vi "PH_VacuumControl.ProcCases.vi"(0 "i ref in":refnum<vi>, 1 "selector":string, 2 "Data":T1, 3 "call cluster":T2={"Object"="", "Selector"="", "CallType"=enum."synchronous", "Async Object"="", "Async Selector"="", "Data Descriptor"="", "Data"=[], "Error #"=0, "Expire"=0}, 5 "error in (no error)":errorcluster) -> (14 "i ref out":refnum<vi>, 17 "answer cluster":T2={"Object"="", "Selector"="", "CallType"=enum."synchronous", "Async Object"="", "Async Selector"="", "Data Descriptor"="", "Data"=[], "Error #"=0, "Expire"=0}, 19 "error out":errorcluster)   [LabVIEW 2014, in "PH_VacuumControl.lvlib"]
doc: "This method is called by a process from within the default case in the event loop. The methods of a class that are linked to events will be called from THIS method. Add your code here."
uses:
  PH_VacuumControl.lvlib
  CSCore/CSSystem/CoreDefs/CoreDefs.call_type.ctl
  CSCore/BaseProcess/BaseProcess.descriptor string definition.ctl
  CSCore/CSSystem/CoreDefs/CoreDefs.rawDataType.ctl
  CSCore/CSSystem/CoreLib/CoreLib.string 2 byte array.vi
  CSCore/CSSystem/CoreLib/CoreLib.byte array 2 double.vi
  CSCore/CSSystem/CoreLib/CoreLib.byte array 2 short.vi
  CSCore/CSSystem/CoreLib/CoreLib.byte array 2 int.vi
  CSCore/CSSystem/CoreLib/CoreLib.lvlib
  CSCore/BaseProcess/BaseProcess.lvlib
  instr.lib/AGCxxx/AGCxxx - Driver.lvlib
  CSCore/CAEObj/CAEObj.lvlib
  PH_PSDBWriter/PH_PSDBWriter.lvlib
  PH_Common/PH_Common.lvlib
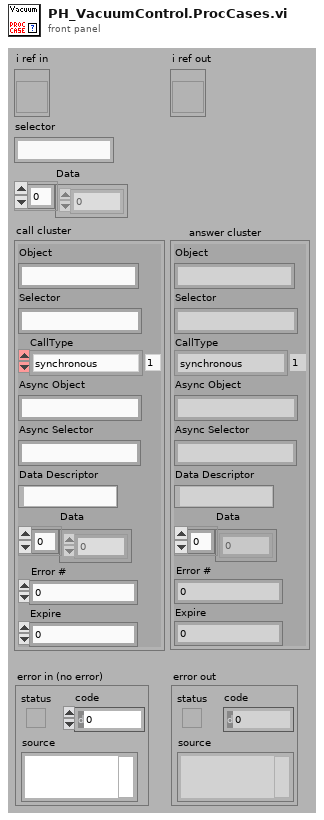
[diagram p1: front panel]
types:
  T1 = typedef "CoreDefs.rawDataType.ctl" = i8[]
  T2 = typedef "CoreDefs.call_type.ctl" = cluster{"Object":string, "Selector":string, "CallType":enum16{"simple", "synchronous", "asynchronous"}, "Async Object":string, "Async Selector":string, "Data Descriptor":T3, "Data":T1, "Error #":i32, "Expire":u32}
  T3 = typedef "BaseProcess.lvlib/BaseProcess.descriptor string definition.ctl" = string
  T4 = typedef "PH_VacuumControl.lvlib/PH_VacuumControl.i attribute.ctl" = cluster{"GUI Refs":cluster{"Exit":refnum<vi>, "Set Unit":refnum<vi>, "Device found":refnum<vi>, "Busy":refnum<vi>, "State":refnum<vi>, "Delete":refnum<vi>, "Channels":refnum<vi>, "Channel Name":refnum<vi>, "Trend":refnum<vi>, "Logarithmic":refnum<vi>, "Limit reached":refnum<vi>, "Channel Name 1 MT":refnum<vi>, "Channel Name 2 MT":refnum<vi>, "Trend MT":refnum<vi>, "Logarithmic MT":refnum<vi>, "Limit reached MT":refnum<vi>}, "Device found":bool, "Busy":bool, "Selected Unit":i32, "Channels [mbar]":T5, "Channel Names":cluster{"Channel 1":string, "Channel 2":string, "Channel 3":string, "Channel 4":string, "Channel 5":string, "Channel 6":string}, "Status":T6, "AGCxxx VISA Cluster":T7, "Instr Firmware Revision":string, "Service IDs Pressure":cluster{"Channel 1":i32, "Channel 2":i32, "Channel 3":i32, "Channel 4":i32, "Channel 5":i32, "Channel 6":i32}, "Service IDs Limits":cluster{"Channel 1":i32, "Channel 2":i32, "Channel 3":i32, "Channel 4":i32, "Channel 5":i32, "Channel 6":i32}, "Trend":cluster{"Start Point":timestamp, "Pressures [mbar] Channel 1":dbl[], "Pressures [mbar] Channel 2":dbl[], "Pressures [mbar] Channel 3":dbl[], "Pressures [mbar] Channel 4":dbl[], "Pressures [mbar] Channel 5":dbl[], "Pressures [mbar] Channel 6":dbl[], "Timebase [s]":i32[], "Trend Channel":u16, "Start Fit":dbl, "Trend Channel 1 MT":u16, "Trend Channel 2 MT":u16, "Start or continue Fit MT":dbl, "Continue or start Fit MT":dbl, "Datasets strored":i32, "Dataarray Size":i32}, "Running":bool}
  T5 = typedef "PH_VacuumControl.lvlib/PH_VacuumControl.Channels.ctl" = cluster{"Channel 1":dbl, "Channel 2":dbl, "Channel 3":dbl, "Channel 4":dbl, "Channel 5":dbl, "Channel 6":dbl, "Name Channel 1":string, "Name Channel 2":string, "Name Channel 3":string, "Name Channel 4":string, "Name Channel 5":string, "Name Channel 6":string, "Upper Limit":dbl, "Upper Limit 2":dbl, "Upper Limit 3":dbl, "Upper Limit 4":dbl, "Upper Limit 5":dbl, "Upper Limit 6":dbl}
  T6 = typedef "PH_StatusHandler.lvlib/PH_StatusHandler.Status.ctl" = i16
  T7 = typedef "AGCxxx - Driver.lvlib/AGCxxx VISA Control.ctl" = cluster{"VISA resource name":refnum<visa-resource-name>, "VISA Timeout Value (1000 ms)":u32, "Lock Timeout (1000 ms)":u32, "MAX Channel (6)":i32}
  T8 = typedef "PH_PSDBWriter.lvlib/PH_PSDBWriter.PHELIX-Subsystems.ctl" = i32
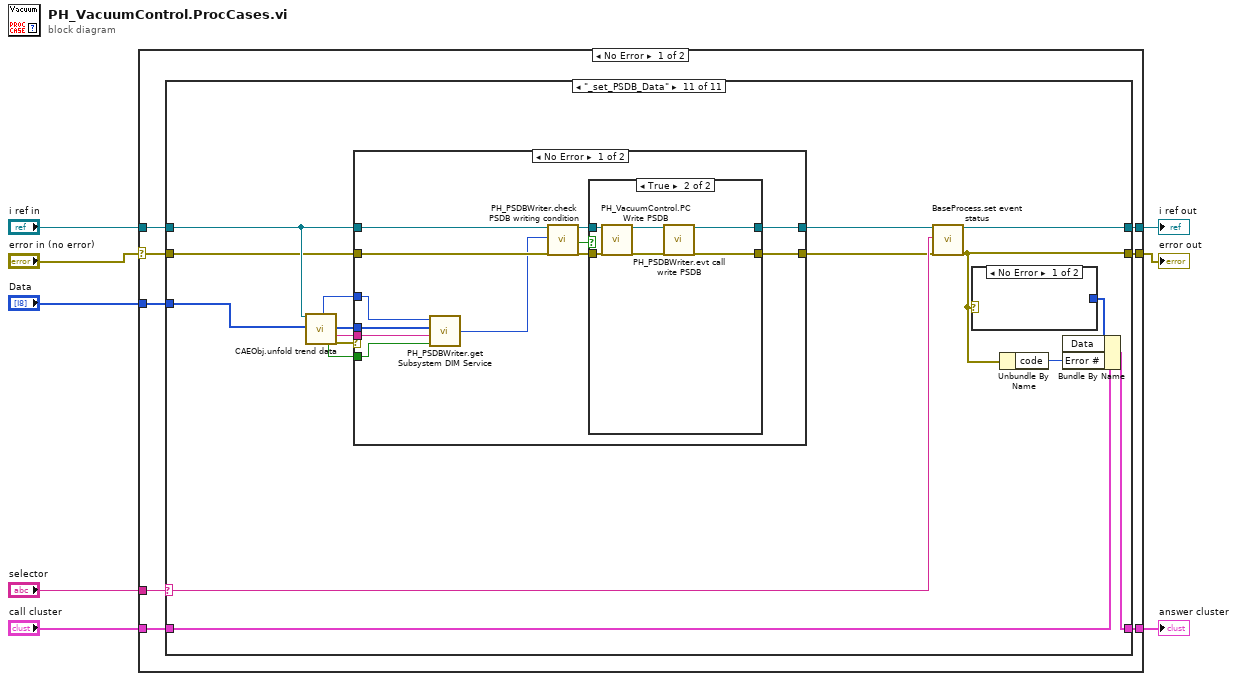
[diagram p0: block diagram]
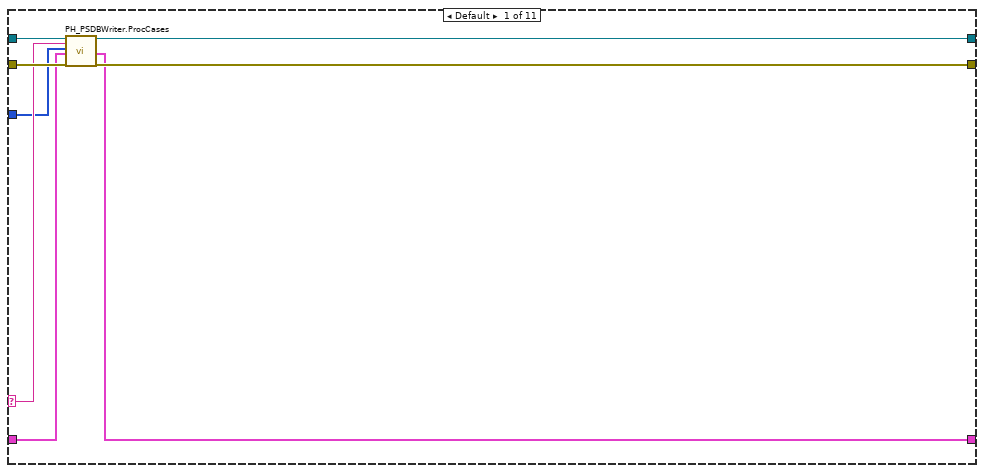
[diagram p2: hidden frame]
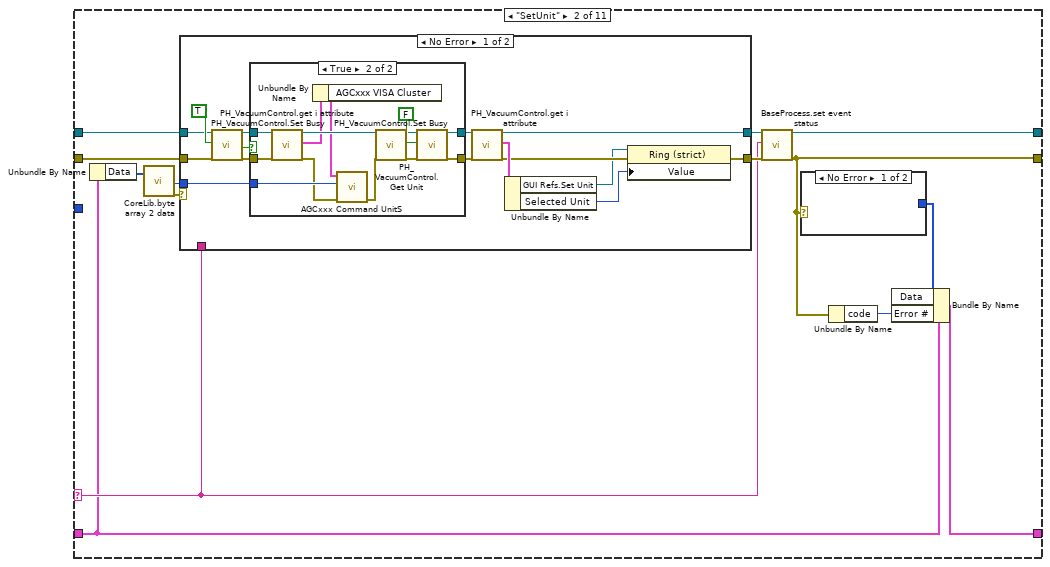
[diagram p3: hidden frame]
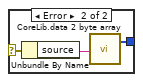
[diagram p4: hidden frame]
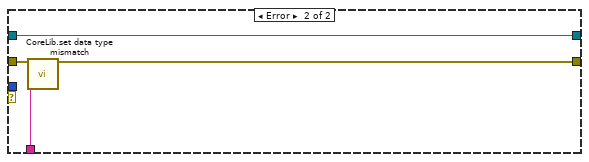
[diagram p6: hidden frame]
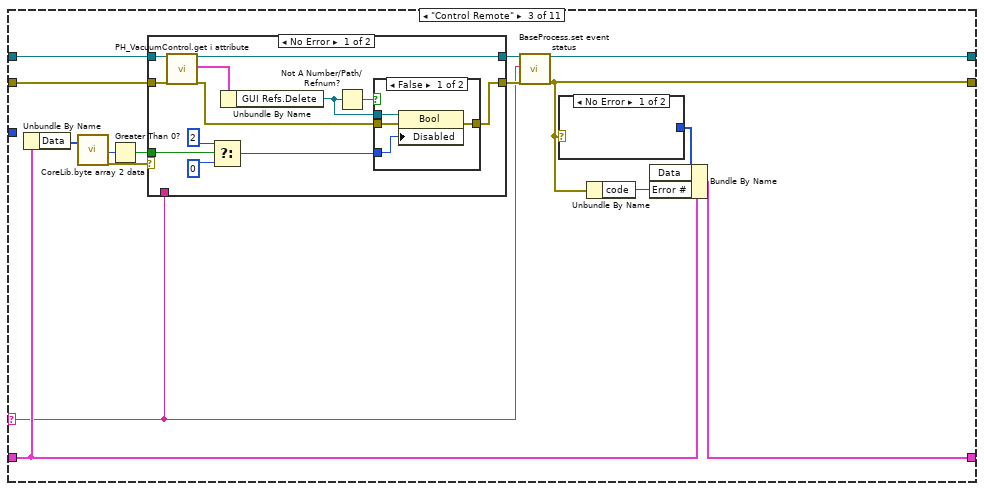
[diagram p7: hidden frame]
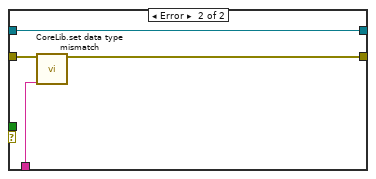
[diagram p9: hidden frame]
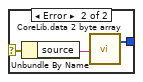
[diagram p10: hidden frame]
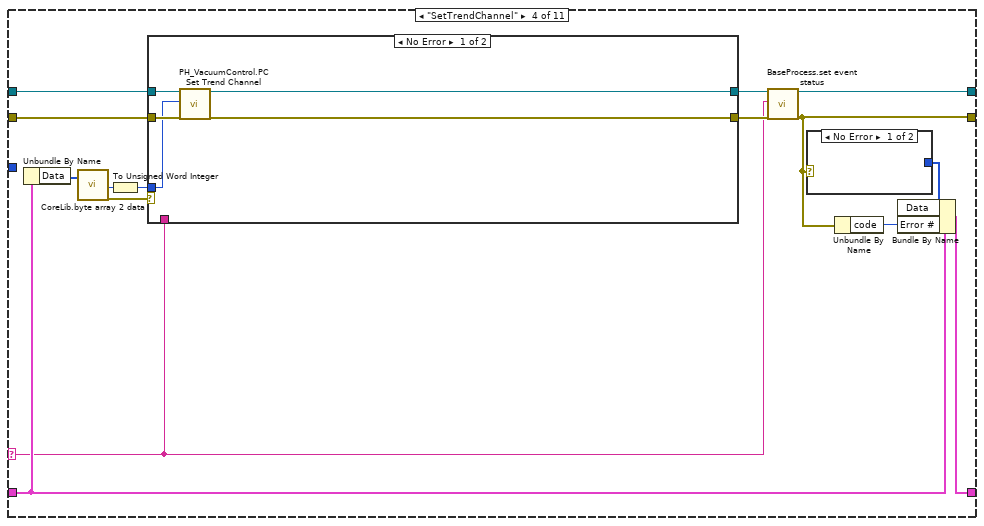
[diagram p11: hidden frame]
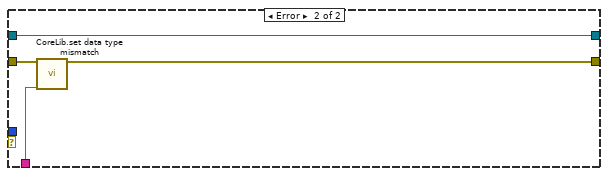
[diagram p12: hidden frame]
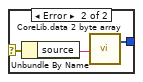
[diagram p13: hidden frame]
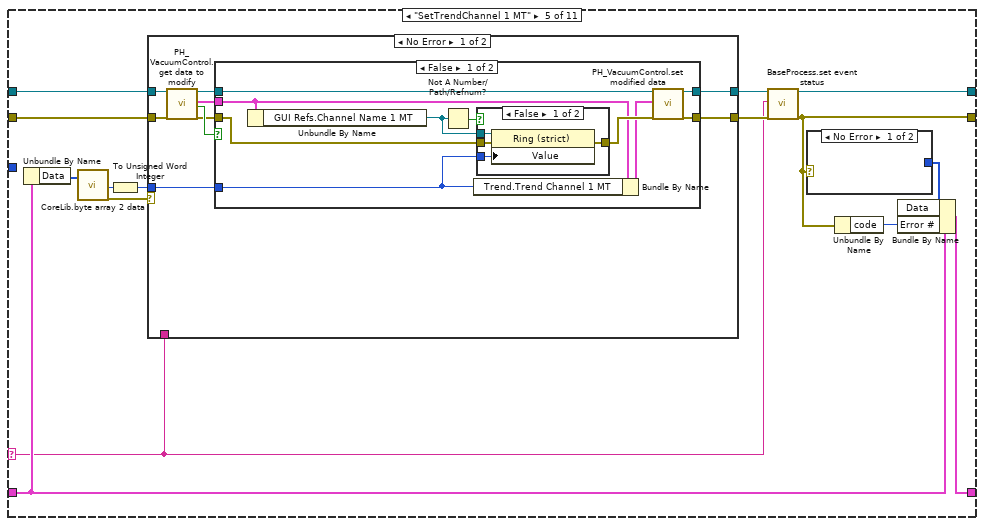
[diagram p14: hidden frame]
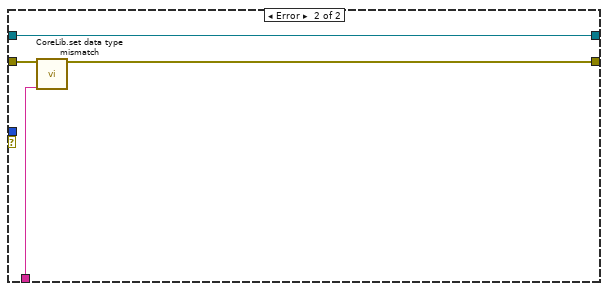
[diagram p17: hidden frame]
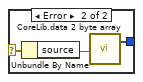
[diagram p18: hidden frame]
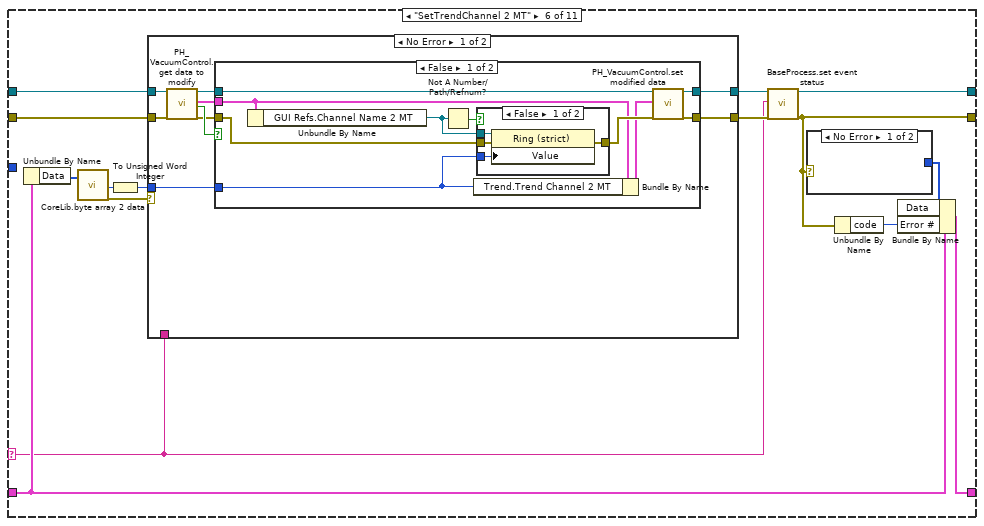
[diagram p19: hidden frame]
diagram:
  n1 = case shown="No Error" "error in (no error)" {
    selector: "error in (no error)" -> [w9 w431]
    tunnel: "selector" -> [w16 _]
    tunnel: [w15 w430] -> w7
    tunnel: "call cluster" -> [w14 w430]
    tunnel: "i ref in" -> [w13 w432]
    tunnel: [w12 w432] -> w4
    tunnel: [w11 w431] -> w3
    tunnel: "Data" -> [w10 _]
    frame No Error {
      n2 = case shown="\"_set_PSDB_Data\"" w16 {
        selector: w16 -> [w19 w27 w77 w116 w143 w191 w240 w267 w306 w349 w398]
        tunnel: w13 -> [w18 w38 w79 w118 w145 w193 w242 w269 w308 w351 w392]
        tunnel: [w24 w29 w88 w127 w154 w202 w250 w277 w316 w358 w402] -> w12
        tunnel: w14 -> [w20 w26 w83 w122 w149 w197 w246 w273 w312 w354 w399]
        tunnel: [w21 w25 w86 w125 w152 w200 w248 w275 w314 w356 w400] -> w15
        tunnel: w9 -> [w23 w37 w81 w120 w147 w195 w244 w271 w310 w353 w391]
        tunnel: [w22 w28 w87 w126 w153 w201 w249 w276 w315 w357 w401] -> w11
        tunnel: w10 -> [w17 _ _ _ _ _ _ _ _ _ w388]
        frame Default {
          n3 = call "PH_PSDBWriter.ProcCases.vi"("i ref in"=w18, "selector"=w19, "Data"=w17, "call cluster"=w20, "error in"=w23) -> ("i ref out"=w24:refnum<vi>, "answer cluster"=w21:T2, "error out"=w22:errorcluster)  [unwired: 12 in]
        }
        frame "SetUnit" {
          n4 = Unbundle By Name(w26) -> ("Data"=w36:T1)
          n5 = call-poly "CoreLib.byte array 2 data.vi"("byteArray"=w36) -> ("i32"=w34:i32, "error out"=w35:errorcluster)  [unwired: 16 in, 1 out]
          n6 = case shown="No Error" w35 {
            tunnel: [w49 w75] -> w30
            tunnel: w38 -> [w51 w75]
            tunnel: w37 -> [w52 w74]
            tunnel: [w44 w73] -> w31
            tunnel: w27 -> [_ w72]
            tunnel: w34 -> [w50 _]
            frame No Error {
              n7 = call "PH_VacuumControl.Set Busy.vi"("i ref in"=w51, "Busy"=TRUE, "error in (no error)"=w52) -> ("i ref out"=w54:refnum<vi>, "changed"=w53:bool, "error out"=w55:errorcluster)  [unwired: 14 in]
              n8 = case shown="True" w53 {
                tunnel: [w57 w70] -> w47
                tunnel: [w58 w69] -> w48
                tunnel: w55 -> [w57 w64]
                tunnel: w54 -> [w58 w66]
                tunnel: w50 -> [_ w61]
                frame False {
                }
                frame True {
                  n9 = call "PH_VacuumControl.get i attribute.vi"("i ref in"=w66, "error in (no error)"=w64) -> ("i ref out"=w65:refnum<vi>, "i attribute"=w63:T4, "error out"=w60:errorcluster)  [unwired: 15 in]
                  n10 = Unbundle By Name(w63) -> ("AGCxxx VISA Cluster"=w62:T7)
                  n11 = call "AGCxxx Command UnitS.vi"("error in (no error)"=w60, "unit (mBar)"=w61, "AGCxxx VISA Cluster"=w62) -> ("error out"=w59:errorcluster)  [unwired: 5 in, 2 out]
                  n12 = call "PH_VacuumControl.Get Unit.vi"("i ref in"=w65, "error in (no error)"=w59) -> ("i ref out"=w68:refnum<vi>, "error out"=w67:errorcluster)  [unwired: 16 in]
                  n13 = call "PH_VacuumControl.Set Busy.vi"("i ref in"=w68, "Busy"=FALSE, "error in (no error)"=w67) -> ("i ref out"=w69:refnum<vi>, "error out"=w70:errorcluster)  [unwired: 14 in, 1 out]
                }
              }
              n14 = call "PH_VacuumControl.get i attribute.vi"("i ref in"=w48, "error in (no error)"=w47) -> ("i ref out"=w49:refnum<vi>, "i attribute"=w46:T4, "error out"=w45:errorcluster)  [unwired: 15 in]
              n15 = Unbundle By Name(w46) -> ("GUI Refs.Set Unit"=w43:refnum<vi>, "Selected Unit"=w42:i32)
              n16 = property class="Ring (strict)"(reference=w43, error in=w45, "Value"=w42) -> (error out=w44:errorcluster)  [unwired: 1 out]
            }
            frame Error {
              n17 = call "CoreLib.set data type mismatch.vi"("error in (no error)"=w74, "error source"=w72) -> ("error out"=w73:errorcluster)  [unwired: 17 in]
            }
          }
          n18 = call "BaseProcess.set event status.vi"("i ref in"=w30, "EventStatus"=w27, "error in (no error)"=w31) -> ("i ref out"=w29:refnum<vi>, "error out"=w28:errorcluster)  [unwired: 14 in, 1 out]
          n19 = case shown="No Error" w28 {
            selector: w28 -> [_ w41]
            tunnel: [_ w39] -> w32
            frame No Error {
            }
            frame Error {
              n20 = Unbundle By Name(w41) -> ("source"=w40:string)
              n21 = call-poly "CoreLib.data 2 byte array.vi"("string"=w40) -> ("byteArray out"=w39:T1)  [unwired: 18 in]
            }
          }
          n22 = Unbundle By Name(w28) -> ("code"=w33:i32)
          n23 = Bundle By Name(cluster=w26, "Data"=w32, "Error #"=w33) -> (w25:T2)
        }
        frame "Control Remote" {
          n24 = Unbundle By Name(w83) -> ("Data"=w85:T1)
          n25 = call-poly "CoreLib.byte array 2 data.vi"("byteArray"=w85) -> ("i16"=w84:i16, "error out"=w82:errorcluster)  [unwired: 16 in, 1 out]
          n26 = Greater Than 0?(x=w84) -> (x > 0?=w76:bool)
          n27 = case shown="No Error" w82 {
            tunnel: w81 -> [w101 w111]
            tunnel: [w98 w110] -> w80
            tunnel: w79 -> [w102 w109]
            tunnel: [w100 w109] -> w78
            tunnel: w77 -> [_ w108]
            tunnel: w76 -> [w94 _]
            frame No Error {
              n28 = call "PH_VacuumControl.get i attribute.vi"("i ref in"=w102, "error in (no error)"=w101) -> ("i ref out"=w100:refnum<vi>, "i attribute"=w99:T4, "error out"=w97:errorcluster)  [unwired: 15 in]
              n29 = Select(t=u8 2 ("Disabled"), s=w94, f=u8 0 ("Disabled")) -> (s? t:f=w93:u8)
              n30 = Unbundle By Name(w99) -> ("GUI Refs.Delete"=w96:refnum<vi>)
              n31 = Not A Number/Path/Refnum?(number/path/refnum=w96) -> (NaN/Path/Refnum?=w95:bool)
              n32 = case shown="False" w95 {
                tunnel: [w106 w107] -> w98
                tunnel: w97 -> [w105 w107]
                tunnel: w96 -> [w104 _]
                tunnel: w93 -> [w103 _]
                frame False {
                  n33 = property class="Bool"(reference=w104, error in=w105, "Disabled"=w103) -> (error out=w106:errorcluster)  [unwired: 1 out]
                }
                frame True {
                }
              }
            }
            frame Error {
              n34 = call "CoreLib.set data type mismatch.vi"("error in (no error)"=w111, "error source"=w108) -> ("error out"=w110:errorcluster)  [unwired: 17 in]
            }
          }
          n35 = call "BaseProcess.set event status.vi"("i ref in"=w78, "EventStatus"=w77, "error in (no error)"=w80) -> ("i ref out"=w88:refnum<vi>, "error out"=w87:errorcluster)  [unwired: 14 in, 1 out]
          n36 = case shown="No Error" w87 {
            selector: w87 -> [_ w114]
            tunnel: [_ w112] -> w89
            frame No Error {
            }
            frame Error {
              n37 = Unbundle By Name(w114) -> ("source"=w113:string)
              n38 = call-poly "CoreLib.data 2 byte array.vi"("string"=w113) -> ("byteArray out"=w112:T1)  [unwired: 18 in]
            }
          }
          n39 = Unbundle By Name(w87) -> ("code"=w90:i32)
          n40 = Bundle By Name(cluster=w83, "Data"=w89, "Error #"=w90) -> (w86:T2)
        }
        frame "SetTrendChannel" {
          n41 = Unbundle By Name(w122) -> ("Data"=w124:T1)
          n42 = call-poly "CoreLib.byte array 2 data.vi"("byteArray"=w124) -> ("i16"=w123:i16, "error out"=w121:errorcluster)  [unwired: 16 in, 1 out]
          n43 = To Unsigned Word Integer(number=w123) -> (unsigned 16bit integer=w115:u16)
          n44 = case shown="No Error" w121 {
            tunnel: w120 -> [w133 w138]
            tunnel: [w132 w137] -> w119
            tunnel: w118 -> [w134 w136]
            tunnel: [w131 w136] -> w117
            tunnel: w116 -> [_ w135]
            tunnel: w115 -> [w130 _]
            frame No Error {
              n45 = call "PH_VacuumControl.PC Set Trend Channel.vi"("i ref in"=w134, "Trend Channel"=w130, "error IO"=w133) -> ("i ref out"=w131:refnum<vi>, "error out"=w132:errorcluster)  [unwired: 15 in]
            }
            frame Error {
              n46 = call "CoreLib.set data type mismatch.vi"("error in (no error)"=w138, "error source"=w135) -> ("error out"=w137:errorcluster)  [unwired: 17 in]
            }
          }
          n47 = call "BaseProcess.set event status.vi"("i ref in"=w117, "EventStatus"=w116, "error in (no error)"=w119) -> ("i ref out"=w127:refnum<vi>, "error out"=w126:errorcluster)  [unwired: 14 in, 1 out]
          n48 = case shown="No Error" w126 {
            selector: w126 -> [_ w141]
            tunnel: [_ w139] -> w128
            frame No Error {
            }
            frame Error {
              n49 = Unbundle By Name(w141) -> ("source"=w140:string)
              n50 = call-poly "CoreLib.data 2 byte array.vi"("string"=w140) -> ("byteArray out"=w139:T1)  [unwired: 18 in]
            }
          }
          n51 = Unbundle By Name(w126) -> ("code"=w129:i32)
          n52 = Bundle By Name(cluster=w122, "Data"=w128, "Error #"=w129) -> (w125:T2)
        }
        frame "SetTrendChannel 1 MT" {
          n53 = Unbundle By Name(w149) -> ("Data"=w151:T1)
          n54 = call-poly "CoreLib.byte array 2 data.vi"("byteArray"=w151) -> ("i16"=w150:i16, "error out"=w148:errorcluster)  [unwired: 16 in, 1 out]
          n55 = To Unsigned Word Integer(number=w150) -> (unsigned 16bit integer=w142:u16)
          n56 = case shown="No Error" w148 {
            tunnel: w147 -> [w160 w186]
            tunnel: [w158 w185] -> w146
            tunnel: w145 -> [w161 w184]
            tunnel: [w159 w184] -> w144
            tunnel: w143 -> [_ w183]
            tunnel: w142 -> [w157 _]
            frame No Error {
              n57 = call "PH_VacuumControl.get data to modify.vi"("i ref in"=w161, "error in (no error)"=w160) -> ("i ref out"=w165:refnum<vi>, "i attribute"=w162:T4, "timed out"=w164:bool, "error out"=w163:errorcluster)  [unwired: 14 in]
              n58 = case shown="False" w164 {
                tunnel: w162 -> [w168 _]
                tunnel: w163 -> [w174 w181]
                tunnel: [w171 w181] -> w158
                tunnel: w165 -> [w170 w182]
                tunnel: [w169 w182] -> w159
                tunnel: w157 -> [w166 _]
                frame False {
                  n59 = Unbundle By Name(w168) -> ("GUI Refs.Channel Name 1 MT"=w173:refnum<vi>)
                  n60 = Not A Number/Path/Refnum?(number/path/refnum=w173) -> (NaN/Path/Refnum?=w172:bool)
                  n61 = Bundle By Name(cluster=w168, "Trend.Trend Channel 1 MT"=w166) -> (w167:T4)
                  n62 = case shown="False" w172 {
                    tunnel: [w179 w180] -> w175
                    tunnel: w174 -> [w178 w180]
                    tunnel: w173 -> [w177 _]
                    tunnel: w166 -> [w176 _]
                    frame False {
                      n63 = property class="Ring (strict)"(reference=w177, error in=w178, "Value"=w176) -> (error out=w179:errorcluster)  [unwired: 1 out]
                    }
                    frame True {
                    }
                  }
                  n64 = call "PH_VacuumControl.set modified data.vi"("i ref in"=w170, "i attribute"=w167, "error in (no error)"=w175) -> ("i ref out"=w169:refnum<vi>, "error out"=w171:errorcluster)  [unwired: 15 in]
                }
                frame True {
                }
              }
            }
            frame Error {
              n65 = call "CoreLib.set data type mismatch.vi"("error in (no error)"=w186, "error source"=w183) -> ("error out"=w185:errorcluster)  [unwired: 17 in]
            }
          }
          n66 = call "BaseProcess.set event status.vi"("i ref in"=w144, "EventStatus"=w143, "error in (no error)"=w146) -> ("i ref out"=w154:refnum<vi>, "error out"=w153:errorcluster)  [unwired: 14 in, 1 out]
          n67 = case shown="No Error" w153 {
            selector: w153 -> [_ w189]
            tunnel: [_ w187] -> w155
            frame No Error {
            }
            frame Error {
              n68 = Unbundle By Name(w189) -> ("source"=w188:string)
              n69 = call-poly "CoreLib.data 2 byte array.vi"("string"=w188) -> ("byteArray out"=w187:T1)  [unwired: 18 in]
            }
          }
          n70 = Unbundle By Name(w153) -> ("code"=w156:i32)
          n71 = Bundle By Name(cluster=w149, "Data"=w155, "Error #"=w156) -> (w152:T2)
        }
        frame "SetTrendChannel 2 MT" {
          n72 = Unbundle By Name(w197) -> ("Data"=w199:T1)
          n73 = call-poly "CoreLib.byte array 2 data.vi"("byteArray"=w199) -> ("i16"=w198:i16, "error out"=w196:errorcluster)  [unwired: 16 in, 1 out]
          n74 = To Unsigned Word Integer(number=w198) -> (unsigned 16bit integer=w190:u16)
          n75 = case shown="No Error" w196 {
            tunnel: w195 -> [w208 w234]
            tunnel: [w206 w233] -> w194
            tunnel: w193 -> [w209 w232]
            tunnel: [w207 w232] -> w192
            tunnel: w191 -> [_ w231]
            tunnel: w190 -> [w205 _]
            frame No Error {
              n76 = call "PH_VacuumControl.get data to modify.vi"("i ref in"=w209, "error in (no error)"=w208) -> ("i ref out"=w213:refnum<vi>, "i attribute"=w210:T4, "timed out"=w212:bool, "error out"=w211:errorcluster)  [unwired: 14 in]
              n77 = case shown="False" w212 {
                tunnel: w210 -> [w216 _]
                tunnel: w211 -> [w222 w229]
                tunnel: [w219 w229] -> w206
                tunnel: w213 -> [w218 w230]
                tunnel: [w217 w230] -> w207
                tunnel: w205 -> [w214 _]
                frame False {
                  n78 = Unbundle By Name(w216) -> ("GUI Refs.Channel Name 2 MT"=w221:refnum<vi>)
                  n79 = Not A Number/Path/Refnum?(number/path/refnum=w221) -> (NaN/Path/Refnum?=w220:bool)
                  n80 = Bundle By Name(cluster=w216, "Trend.Trend Channel 2 MT"=w214) -> (w215:T4)
                  n81 = case shown="False" w220 {
                    tunnel: [w227 w228] -> w223
                    tunnel: w222 -> [w226 w228]
                    tunnel: w221 -> [w225 _]
                    tunnel: w214 -> [w224 _]
                    frame False {
                      n82 = property class="Ring (strict)"(reference=w225, error in=w226, "Value"=w224) -> (error out=w227:errorcluster)  [unwired: 1 out]
                    }
                    frame True {
                    }
                  }
                  n83 = call "PH_VacuumControl.set modified data.vi"("i ref in"=w218, "i attribute"=w215, "error in (no error)"=w223) -> ("i ref out"=w217:refnum<vi>, "error out"=w219:errorcluster)  [unwired: 15 in]
                }
                frame True {
                }
              }
            }
            frame Error {
              n84 = call "CoreLib.set data type mismatch.vi"("error in (no error)"=w234, "error source"=w231) -> ("error out"=w233:errorcluster)  [unwired: 17 in]
            }
          }
          n85 = call "BaseProcess.set event status.vi"("i ref in"=w192, "EventStatus"=w191, "error in (no error)"=w194) -> ("i ref out"=w202:refnum<vi>, "error out"=w201:errorcluster)  [unwired: 14 in, 1 out]
          n86 = case shown="No Error" w201 {
            selector: w201 -> [_ w237]
            tunnel: [_ w235] -> w203
            frame No Error {
            }
            frame Error {
              n87 = Unbundle By Name(w237) -> ("source"=w236:string)
              n88 = call-poly "CoreLib.data 2 byte array.vi"("string"=w236) -> ("byteArray out"=w235:T1)  [unwired: 18 in]
            }
          }
          n89 = Unbundle By Name(w201) -> ("code"=w204:i32)
          n90 = Bundle By Name(cluster=w197, "Data"=w203, "Error #"=w204) -> (w200:T2)
        }
        frame "SetLogarithmic" {
          n91 = Unbundle By Name(w246) -> ("Data"=w247:T1)
          n92 = call-poly "CoreLib.byte array 2 data.vi"("byteArray"=w247) -> ("i16"=w239:i16, "error out"=w245:errorcluster)  [unwired: 16 in, 1 out]
          n93 = Greater Than 0?(x=w239) -> (x > 0?=w238:bool)
          n94 = case shown="No Error" w245 {
            tunnel: w244 -> [w256 w261]
            tunnel: [w254 w260] -> w243
            tunnel: w242 -> [w257 w259]
            tunnel: [w255 w259] -> w241
            tunnel: w240 -> [_ w258]
            tunnel: w238 -> [w253 _]
            frame No Error {
              n95 = call "PH_VacuumControl.PC Set Logarithmic.vi"("i ref in"=w257, "Logarithmic"=w253, "error IO"=w256) -> ("i ref out"=w255:refnum<vi>, "error out"=w254:errorcluster)  [unwired: 15 in]
            }
            frame Error {
              n96 = call "CoreLib.set data type mismatch.vi"("error in (no error)"=w261, "error source"=w258) -> ("error out"=w260:errorcluster)  [unwired: 17 in]
            }
          }
          n97 = call "BaseProcess.set event status.vi"("i ref in"=w241, "EventStatus"=w240, "error in (no error)"=w243) -> ("i ref out"=w250:refnum<vi>, "error out"=w249:errorcluster)  [unwired: 14 in, 1 out]
          n98 = case shown="No Error" w249 {
            selector: w249 -> [_ w264]
            tunnel: [_ w262] -> w251
            frame No Error {
            }
            frame Error {
              n99 = Unbundle By Name(w264) -> ("source"=w263:string)
              n100 = call-poly "CoreLib.data 2 byte array.vi"("string"=w263) -> ("byteArray out"=w262:T1)  [unwired: 18 in]
            }
          }
          n101 = Unbundle By Name(w249) -> ("code"=w252:i32)
          n102 = Bundle By Name(cluster=w246, "Data"=w251, "Error #"=w252) -> (w248:T2)
        }
        frame "SetMTLogarithmic" {
          n103 = Unbundle By Name(w273) -> ("Data"=w274:T1)
          n104 = call-poly "CoreLib.byte array 2 data.vi"("byteArray"=w274) -> ("i16"=w266:i16, "error out"=w272:errorcluster)  [unwired: 16 in, 1 out]
          n105 = Greater Than 0?(x=w266) -> (x > 0?=w265:bool)
          n106 = case shown="No Error" w272 {
            tunnel: w271 -> [w284 w301]
            tunnel: [w281 w300] -> w270
            tunnel: w269 -> [w283 w299]
            tunnel: [w282 w299] -> w268
            tunnel: w267 -> [_ w298]
            tunnel: w265 -> [w280 _]
            frame No Error {
              n107 = call "PH_VacuumControl.get i attribute.vi"("i ref in"=w283, "error in (no error)"=w284) -> ("i ref out"=w282:refnum<vi>, "i attribute"=w287:T4, "error out"=w288:errorcluster)  [unwired: 15 in]
              n108 = Unbundle By Name(w287) -> ("GUI Refs.Logarithmic MT"=w292:refnum<vi>, "GUI Refs.Trend MT"=w289:refnum<vi>)
              n109 = Boolean To (0,1)(Boolean=w280) -> (0, 1=w286:i16)
              n110 = To Unsigned Byte Integer(number=w286) -> (unsigned 8bit integer=w285:u8)
              n111 = Not A Number/Path/Refnum?(number/path/refnum=w289) -> (NaN/Path/Refnum?=w290:bool)
              n112 = case shown="False" w290 {
                tunnel: w285 -> [w296 _]
                tunnel: w289 -> [w295 _]
                tunnel: w288 -> [w294 w297]
                tunnel: [w293 w297] -> w291
                frame False {
                  n113 = property class="XYGraph (strict)"(reference=w295, error in=w294, "YScale.Mapping Mode"=w296) -> (error out=w293:errorcluster)  [unwired: 1 out]
                }
                frame True {
                }
              }
              n114 = call "PH_GUI.set boolean GUI object.vi"("Boolean Knob GUI Ref"=w292, "Value"=w280, "error in (no error)"=w291) -> ("error out"=w281:errorcluster)  [unwired: 16 in]
            }
            frame Error {
              n115 = call "CoreLib.set data type mismatch.vi"("error in (no error)"=w301, "error source"=w298) -> ("error out"=w300:errorcluster)  [unwired: 17 in]
            }
          }
          n116 = call "BaseProcess.set event status.vi"("i ref in"=w268, "EventStatus"=w267, "error in (no error)"=w270) -> ("i ref out"=w277:refnum<vi>, "error out"=w276:errorcluster)  [unwired: 14 in, 1 out]
          n117 = case shown="No Error" w276 {
            selector: w276 -> [_ w304]
            tunnel: [_ w302] -> w278
            frame No Error {
            }
            frame Error {
              n118 = Unbundle By Name(w304) -> ("source"=w303:string)
              n119 = call-poly "CoreLib.data 2 byte array.vi"("string"=w303) -> ("byteArray out"=w302:T1)  [unwired: 18 in]
            }
          }
          n120 = Unbundle By Name(w276) -> ("code"=w279:i32)
          n121 = Bundle By Name(cluster=w273, "Data"=w278, "Error #"=w279) -> (w275:T2)
        }
        frame "SetFitStart" {
          n122 = Unbundle By Name(w312) -> ("Data"=w313:T1)
          n123 = call-poly "CoreLib.byte array 2 data.vi"("byteArray"=w313) -> ("d64"=w305:dbl, "error out"=w311:errorcluster)  [unwired: 16 in, 1 out]
          n124 = case shown="No Error" w311 {
            tunnel: w310 -> [w326 w340]
            tunnel: [w322 w339] -> w309
            tunnel: w308 -> [w327 w338]
            tunnel: [w324 w338] -> w307
            tunnel: w306 -> [_ w337]
            tunnel: w305 -> [w319 _]
            frame No Error {
              n125 = call "PH_VacuumControl.get data to modify.vi"("i ref in"=w327, "error in (no error)"=w326) -> ("i ref out"=w325:refnum<vi>, "i attribute"=w320:T4, "timed out"=w321:bool, "error out"=w323:errorcluster)  [unwired: 14 in]
              n126 = case shown="False" w321 {
                tunnel: w325 -> [w334 w336]
                tunnel: [w333 w336] -> w324
                tunnel: w323 -> [w332 w335]
                tunnel: [w331 w335] -> w322
                tunnel: w320 -> [w330 _]
                tunnel: w319 -> [w328 _]
                frame False {
                  n127 = Bundle By Name(cluster=w330, "Trend.Start Fit"=w328) -> (w329:T4)
                  n128 = call "PH_VacuumControl.set modified data.vi"("i ref in"=w334, "i attribute"=w329, "error in (no error)"=w332) -> ("i ref out"=w333:refnum<vi>, "error out"=w331:errorcluster)  [unwired: 15 in]
                }
                frame True {
                }
              }
            }
            frame Error {
              n129 = call "CoreLib.set data type mismatch.vi"("error in (no error)"=w340, "error source"=w337) -> ("error out"=w339:errorcluster)  [unwired: 17 in]
            }
          }
          n130 = call "BaseProcess.set event status.vi"("i ref in"=w307, "EventStatus"=w306, "error in (no error)"=w309) -> ("i ref out"=w316:refnum<vi>, "error out"=w315:errorcluster)  [unwired: 14 in, 1 out]
          n131 = case shown="No Error" w315 {
            selector: w315 -> [_ w343]
            tunnel: [_ w341] -> w317
            frame No Error {
            }
            frame Error {
              n132 = Unbundle By Name(w343) -> ("source"=w342:string)
              n133 = call-poly "CoreLib.data 2 byte array.vi"("string"=w342) -> ("byteArray out"=w341:T1)  [unwired: 18 in]
            }
          }
          n134 = Unbundle By Name(w315) -> ("code"=w318:i32)
          n135 = Bundle By Name(cluster=w312, "Data"=w317, "Error #"=w318) -> (w314:T2)
        }
        frame "SetFitStart MT" {
          n136 = Unbundle By Name(w354) -> ("Data"=w355:T1)
          n137 = call-poly "CoreLib.byte array 2 data.vi"("byteArray"=w355) -> ("byteArray out"=w345:T1, "d64"=w348:dbl, "error out"=w347:errorcluster)  [unwired: 16 in]
          n138 = call-poly "CoreLib.byte array 2 data.vi"("byteArray"=w345, "error in (no error)"=w347) -> ("d64"=w344:dbl, "error out"=w346:errorcluster)  [unwired: 15 in, 1 out]
          n139 = case shown="No Error" w346 {
            tunnel: w353 -> [w369 w384]
            tunnel: [w367 w383] -> w352
            tunnel: w351 -> [w370 w382]
            tunnel: [w368 w382] -> w350
            tunnel: w349 -> [_ w381]
            tunnel: w348 -> [w366 _]
            tunnel: w344 -> [w361 _]
            frame No Error {
              n140 = call "PH_VacuumControl.get data to modify.vi"("i ref in"=w370, "error in (no error)"=w369) -> ("i ref out"=w365:refnum<vi>, "i attribute"=w362:T4, "timed out"=w363:bool, "error out"=w364:errorcluster)  [unwired: 14 in]
              n141 = case shown="False" w363 {
                tunnel: w365 -> [w378 w380]
                tunnel: [w377 w380] -> w368
                tunnel: w364 -> [w376 w379]
                tunnel: [w375 w379] -> w367
                tunnel: w362 -> [w374 _]
                tunnel: w366 -> [w372 _]
                tunnel: w361 -> [w371 _]
                frame False {
                  n142 = Bundle By Name(cluster=w374, "Trend.Start or continue Fit MT"=w372, "Trend.Continue or start Fit MT"=w371) -> (w373:T4)
                  n143 = call "PH_VacuumControl.set modified data.vi"("i ref in"=w378, "i attribute"=w373, "error in (no error)"=w376) -> ("i ref out"=w377:refnum<vi>, "error out"=w375:errorcluster)  [unwired: 15 in]
                }
                frame True {
                }
              }
            }
            frame Error {
              n144 = call "CoreLib.set data type mismatch.vi"("error in (no error)"=w384, "error source"=w381) -> ("error out"=w383:errorcluster)  [unwired: 17 in]
            }
          }
          n145 = call "BaseProcess.set event status.vi"("i ref in"=w350, "EventStatus"=w349, "error in (no error)"=w352) -> ("i ref out"=w358:refnum<vi>, "error out"=w357:errorcluster)  [unwired: 14 in, 1 out]
          n146 = case shown="No Error" w357 {
            selector: w357 -> [_ w387]
            tunnel: [_ w385] -> w359
            frame No Error {
            }
            frame Error {
              n147 = Unbundle By Name(w387) -> ("source"=w386:string)
              n148 = call-poly "CoreLib.data 2 byte array.vi"("string"=w386) -> ("byteArray out"=w385:T1)  [unwired: 18 in]
            }
          }
          n149 = Unbundle By Name(w357) -> ("code"=w360:i32)
          n150 = Bundle By Name(cluster=w354, "Data"=w359, "Error #"=w360) -> (w356:T2)
        }
        frame "_set_PSDB_Data" {
          n151 = call "CAEObj.unfold trend data.vi"("i ref in"=w392, "raw trend data"=w388) -> ("quality"=w393:i32, "no link"=w396:bool, "data"=w394:i8[], "typeDescriptor"=w395:string, "error out"=w397:errorcluster)  [unwired: 9 in, 4 out]
          n152 = case shown="No Error" w397 {
            tunnel: w391 -> [w416 w426]
            tunnel: [w415 w425] -> w390
            tunnel: [w414 w426] -> w389
            tunnel: w392 -> [w412 w425]
            tunnel: w396 -> [w407 _]
            tunnel: w395 -> [w408 _]
            tunnel: w394 -> [w409 _]
            tunnel: w393 -> [w406 _]
            frame No Error {
              n153 = call "PH_PSDBWriter.get Subsystem DIM Service.vi"("no link"=w407, "typeDescriptor"=w408, "data"=w409, "quality"=w406) -> ("PHELIX Subsystems"=w405:T8)
              n154 = call "PH_PSDBWriter.check PSDB writing condition.vi"("i ref in"=w412, "wanted Subsystem"=w405, "error IO"=w416) -> ("i ref out"=w411:refnum<vi>, "write PSDB?"=w410:bool, "error out"=w413:errorcluster)  [unwired: 14 in]
              n155 = case shown="True" w410 {
                tunnel: w413 -> [w417 w424]
                tunnel: [w418 w421] -> w415
                tunnel: [w417 w419] -> w414
                tunnel: w411 -> [w418 w423]
                frame False {
                }
                frame True {
                  n156 = call "PH_VacuumControl.PC Write PSDB.vi"("i ref in"=w423, "error IO"=w424) -> ("i ref out"=w422:refnum<vi>, "error out"=w420:errorcluster)  [unwired: 16 in]
                  n157 = call "PH_PSDBWriter.evt call write PSDB.vi"("i ref in"=w422, "error in (no error)"=w420) -> ("i ref out"=w421:refnum<vi>, "error out"=w419:errorcluster)  [unwired: 16 in]
                }
              }
            }
            frame Error {
            }
          }
          n158 = call "BaseProcess.set event status.vi"("i ref in"=w390, "EventStatus"=w398, "error in (no error)"=w389) -> ("i ref out"=w402:refnum<vi>, "error out"=w401:errorcluster)  [unwired: 14 in, 1 out]
          n159 = case shown="No Error" w401 {
            selector: w401 -> [_ w429]
            tunnel: [_ w427] -> w403
            frame No Error {
            }
            frame Error {
              n160 = Unbundle By Name(w429) -> ("source"=w428:string)
              n161 = call-poly "CoreLib.data 2 byte array.vi"("string"=w428) -> ("byteArray out"=w427:T1)  [unwired: 18 in]
            }
          }
          n162 = Unbundle By Name(w401) -> ("code"=w404:i32)
          n163 = Bundle By Name(cluster=w399, "Data"=w403, "Error #"=w404) -> (w400:T2)
        }
      }
    }
    frame Error {
    }
  }
  "answer cluster" <- w7
  "i ref out" <- w4
  "error out" <- w3
